vi "RDS Serial Handle Frame.vi"(8 "error in (no error)":errorcluster, 10 "RDS Serial Frame":refnum<class "RDS Serial Frame.lvclass">, 11 "Compass Instrument in":refnum<class "Compass Instrument.lvclass">) -> (0 "error out":errorcluster, 3 "Compass Instrument out":refnum<class "Compass Instrument.lvclass">)   [LabVIEW 2015, in "Compass Instrument.lvlib" / "Compass Instrument.lvclass"]
uses:
  Compass Instrument.lvclass
  RDS Serial Handler/RDS Serial Frame.lvclass
  Actors/RDS Parent Actor/RDS Parent Actor/RDS Parent Actor.lvclass
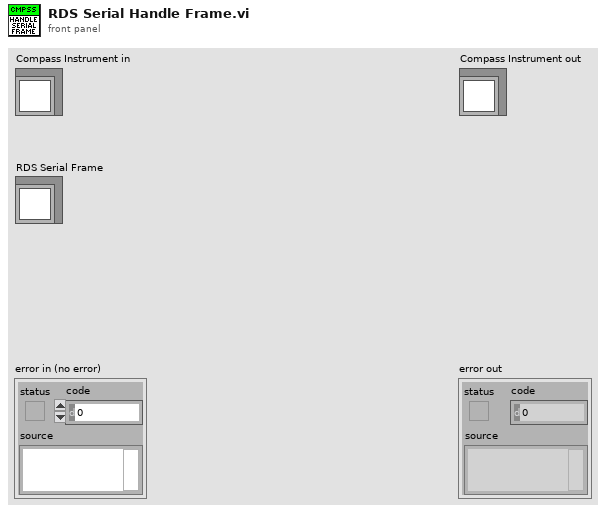
[diagram p1: front panel]
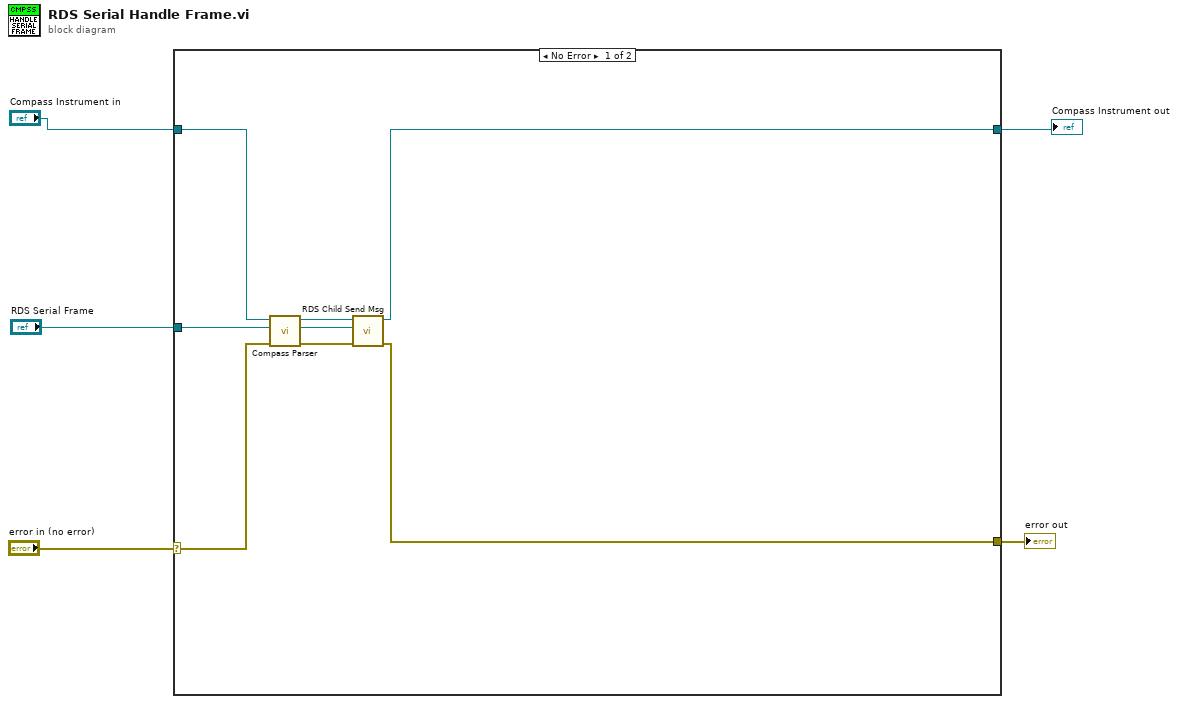
[diagram p0: block diagram]
diagram:
  n1 = case shown="No Error" "error in (no error)" {
    selector: "error in (no error)" -> [w6 w14]
    tunnel: "RDS Serial Frame" -> [w9 _]
    tunnel: "Compass Instrument in" -> [w10 w15]
    tunnel: [w12 w15] -> w2
    tunnel: [w13 w14] -> w1
    frame No Error {
      n2 = call "Compass Parser.vi"("error in (no error)"=w6, "RDS Serial Frame"=w9, "Compass Instrument in"=w10) -> ("error out"=w7:errorcluster, "RDS Message out"=w8:refnum<class "Compass Data Message.lvclass">, "Compass Instrument out"=w11:refnum<class "Compass Instrument.lvclass">)  [unwired: 6 in]
      n3 = call "RDS Child Send Msg.vi"("error in (no error)"=w7, "RDS Message"=w8, "RDS Parent Actor in"=w11) -> ("error out"=w13:errorcluster, "RDS Parent Actor out"=w12:refnum<class "Compass Instrument.lvclass">)  [unwired: 7 in]
    }
    frame Error {
    }
  }
  "error out" <- w1
  "Compass Instrument out" <- w2
